vi "Set Elevation Angle.vi"(8 "error in (no error)":errorcluster, 10 "ElevationAngle":i32 min=-27 max=27, 11 "Kinect Session in":refnum<class "Kinect Session.lvclass">) -> (0 "error out":errorcluster, 2 "Success?":bool, 3 "Kinect Session out":refnum<class "Kinect Session.lvclass">)   [LabVIEW 2014, in "Kinect Library.lvlib"]
doc: "This VI will adjust the angle of the Kinect motor in the vertical axis. If the value is out of range, it is coerced to the Max or Min Values. These Max and Min Values can be obtained using the Get Device Info VI. This funtion will block until the operation is complete."
uses:
  Kinect Library.lvlib
  Kinect Session.lvclass
  Microsoft.Kinect
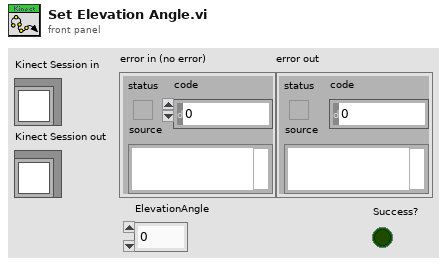
[diagram p1: front panel]
types:
  T1 = cluster{"status":bool, "code":bool, "source":bool}
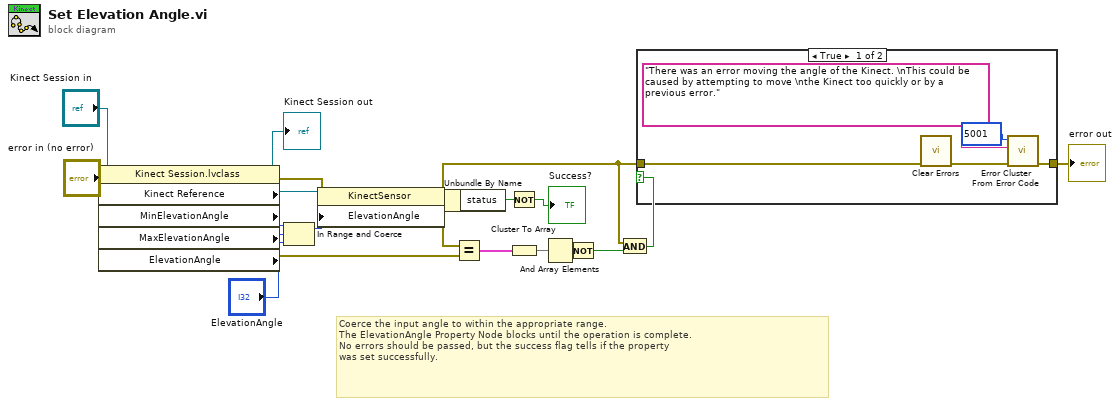
[diagram p0: block diagram]
diagram:
  # "Coerce the input angle to within the appropriate range.\nThe ElevationAngle Property Node blocks until the operation is complete.\nNo errors should be passed, but the success flag tells if the property\nwas set successfully."
  n1 = property class="Kinect Session.lvclass" props=["Kinect Reference", "MinElevationAngle", "MaxElevationAngle", "ElevationAngle"](reference="Kinect Session in", error in="error in (no error)") -> (reference out=→"Kinect Session out":refnum<class "Kinect Session.lvclass">, error out=w15:errorcluster, "Kinect Reference"=w16:refnum<k24>, "MinElevationAngle"=w10:i32, "MaxElevationAngle"=w11:i32)  [unwired: 1 out]
  n2 = In Range and Coerce(upper limit=w11, x="ElevationAngle", lower limit=w10) -> (coerced(x)=w9:i32)  [unwired: 1 out]
  n3 = property class="KinectSensor"(reference=w16, error in=w15, "ElevationAngle"=w9) -> (error out=w2:errorcluster)  [unwired: 1 out]
  n4 = Unbundle By Name(w2) -> ("status"=w14:bool)
  n5 = Equal?(x=w2, y="error in (no error)") -> (x = y?=w6:T1)
  n6 = Not(x=w14) -> (.not. x?=→"Success?":bool)
  n7 = Cluster To Array(cluster=w6) -> (array=w5:bool[])
  n8 = And Array Elements(Boolean array=w5) -> (logical AND=w4:bool)
  n9 = Not(x=w4) -> (.not. x?=w1:bool)
  n10 = And(x=w2, y=w1) -> (x .and. y?=w3:bool)
  n11 = case shown="True" w3 {
    tunnel: [w23 w24] -> w8
    tunnel: w2 -> [w20 w24]
    frame True {
      n12 = call <vilib>:"Clear Errors.vi"("error in (no error)"=w20) -> ("error out"=w19:errorcluster)  [unwired: 5 in, 1 out]
      n13 = call <vilib>:"Error Cluster From Error Code.vi"("error in (no error)"=w19, "error message (\"\")"="There was an error moving the angle of the Kinect. \nThis could be caused by attempting to move \nthe Kinect too quickly or by a previous error." ("error message (\"\")"), "error code (0)"=5001) -> ("error out"=w23:errorcluster)  [unwired: 6 in]
    }
    frame False {
    }
  }
  "error out" <- w8
